vi "UDP Multicast-Server.vi"() -> ()   [LabVIEW 2019]
doc: "Creates a write-only UDP multicast session and sends data to the specified port."
uses:
  <vilib>/Utility/tcp.llb/UDP Multicast Write-Only Open.vi
panel:
  out "Current Data Value":dbl
  in  "Stop":bool
  # "Overview: Demonstrates the use of the UDP functions to initialize a UDP multicast session for sending data.\nInstructions:\n1. Run the VI.\n2. Open UDP Multicast - Receiver.vi and follow the instructions on its front panel.\n3. Click Stop to stop the VI."
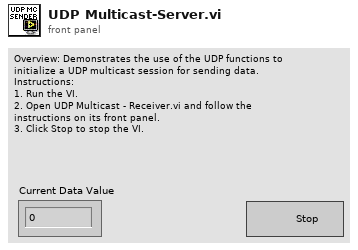
[diagram p1: front panel]
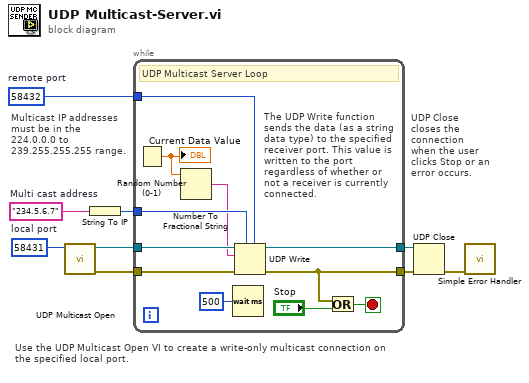
[diagram p0: block diagram]
diagram:
  w1 = u16 58432  # remote port
  w2 = u16 58431  # local port
  w7 = "234.5.6.7"  # Multi cast address
  # "UDP Close closes the connection when the user clicks Stop or an error occurs."
  # "Multicast IP addresses must be in the 224.0.0.0 to 239.255.255.255 range."
  # "Use the UDP Multicast Open VI to create a write-only multicast connection on the specified local port."
  n1 = call-poly <vilib>:"UDP Multicast Open.vi"("port"=w2) -> ("error out"=w3:errorcluster, "connection ID"=w4:refnum<k16>)  [unwired: 9 in]
  n2 = String To IP(1:w7) -> (0:w5:u32)
  n3 = while {
    tunnel: [w15] -> w8
    tunnel: w4 -> [w20]
    tunnel: w3 -> [w19]
    tunnel: [w16] -> w9
    tunnel: w5 -> [w14]
    tunnel: w1 -> [w11]
    stop <- w18 stop-if-true
    # "The UDP Write function sends the data (as a string data type) to the specified receiver port. This value is written to the port regardless of whether or not a receiver is currently connected."
    # "UDP Multicast Server Loop"
    n4 = Random Number (0-1)() -> (number: 0 to 1=w10:dbl)
    "Current Data Value" <- w10
    n5 = Number To Fractional String(number=w10) -> (F-format string=w12:string)  [unwired: 3 in]
    n6 = Wait (ms)(milliseconds to wait=u32 500) -> ()  [unwired: 1 out]
    n7 = UDP Write(address=w14, port or service name=w11, connection ID=w20, data in=w12, 8:w19) -> (error out=w15:errorcluster, 3:w16:refnum<k16>)  [unwired: 1 in]
    n8 = Or(x=w15, y="Stop") -> (x .or. y?=w18:bool)
  }
  n9 = UDP Close(connection ID=w9, 8:w8) -> (error out=w6:errorcluster)  [unwired: 1 out]
  n10 = call <vilib>:"Simple Error Handler.vi"("error in (no error)"=w6) -> ()  [unwired: 4 in, 5 out]
